vi "Test.vi"() -> ()   [LabVIEW 2020]
uses:
  Classes/KD Tree/KD Tree.lvclass
  Classes/KD Tree Double/Create KD Tree Double.vi
  Classes/KD Tree Double/KD Tree Double.lvclass
  <vilib>/Analysis/NI_AALBase.lvlib
  Classes/KD Tree Double/Find Nearest Neighbors Index Double.vi
  E:/Labview/LV 2020/Schmiedeteilvermessung/Source/libs/SK Spatial/flann/Classes/KD Tree/KD Tree.lvclass
  E:/Labview/LV 2020/Schmiedeteilvermessung/Source/libs/SK Spatial/flann/Classes/KD Tree Double/KD Tree Double.lvclass
  Classes/KD Tree Double/Radius Search Double.vi
  <vilib>/numeric/Random Number (Range) I64.vi
  <vilib>/Analysis/baseanly.llb/Mean (DBL).vi
  flann/Flann Params.ctl
  KD Tree.lvlib
panel:
  out "x/y":dbl
  out "mean":dbl format="%0.2f"
  in  "flann_params 2":T1={"algorithm"=0, "checks"=0, "eps"=0.0, "sorted"=1, "max_neighbors"=-1, "cores"=0, "trees"=0, "leaf_max_size"=0, "branching"=0, "iterations"=0, "centers_init"=0, "cb_index"=0.0, "target_precision"=0.0, "build_weight"=0.0, "memory_weight"=0.0, "sample_fraction"=0.0, "table_number_"=0, "key_size_"=0, "multi_probe_level_"=0, "log_level"=0, "random_seed"=0} {"algorithm" items=["FLANN_INDEX_LINEAR"=0, "FLANN_INDEX_KDTREE"=1, "FLANN_INDEX_KMEANS"=2, "FLANN_INDEX_COMPOSITE"=3, "FLANN_INDEX_KDTREE_SINGLE"=4, "FLANN_INDEX_HIERARCHICAL"=5, "FLANN_INDEX_LSH"=6, "FLANN_INDEX_SAVED"=254, "FLANN_INDEX_AUTOTUNED"=255]; "centers_init" items=["FLANN_CENTERS_RANDOM", "FLANN_CENTERS_GONZALES", "FLANN_CENTERS_KMEANSPP", "FLANN_CENTERS_GROUPWISE"]; "log_level" items=["FLANN_LOG_NONE", "FLANN_LOG_FATAL", "FLANN_LOG_ERROR", "FLANN_LOG_WARN", "FLANN_LOG_INFO", "FLANN_LOG_DEBUG"]}
  out "Ref 2":u64
  out "Ref":u64
  out "P4":dbl[][](array[numeric])
  out "Array":dbl[](array[numeric])
  out "Histogram Graph":T2(graph)
  out "P1":dbl[][](array[numeric])
  out "P2":dbl[][](array[numeric])
  out "Intensity Graph":dbl[][](graph)
  in  "flann_params":T1={"algorithm"=0, "checks"=0, "eps"=0.0, "sorted"=1, "max_neighbors"=-1, "cores"=0, "trees"=0, "leaf_max_size"=0, "branching"=0, "iterations"=0, "centers_init"=0, "cb_index"=0.0, "target_precision"=0.0, "build_weight"=0.0, "memory_weight"=0.0, "sample_fraction"=0.0, "table_number_"=0, "key_size_"=0, "multi_probe_level_"=0, "log_level"=0, "random_seed"=0} {"algorithm" items=["FLANN_INDEX_LINEAR"=0, "FLANN_INDEX_KDTREE"=1, "FLANN_INDEX_KMEANS"=2, "FLANN_INDEX_COMPOSITE"=3, "FLANN_INDEX_KDTREE_SINGLE"=4, "FLANN_INDEX_HIERARCHICAL"=5, "FLANN_INDEX_LSH"=6, "FLANN_INDEX_SAVED"=254, "FLANN_INDEX_AUTOTUNED"=255]; "centers_init" items=["FLANN_CENTERS_RANDOM", "FLANN_CENTERS_GONZALES", "FLANN_CENTERS_KMEANSPP", "FLANN_CENTERS_GROUPWISE"]; "log_level" items=["FLANN_LOG_NONE", "FLANN_LOG_FATAL", "FLANN_LOG_ERROR", "FLANN_LOG_WARN", "FLANN_LOG_INFO", "FLANN_LOG_DEBUG"]}
  out "error out":errorcluster
  out "N Found":i32[](array[numeric])
  out "Dists 2":dbl[][](array[numeric])
  out "Indices 2":i32[][](array[numeric])
  out "Dists":dbl[][](array[numeric])
  out "Indices":i32[][](array[numeric])
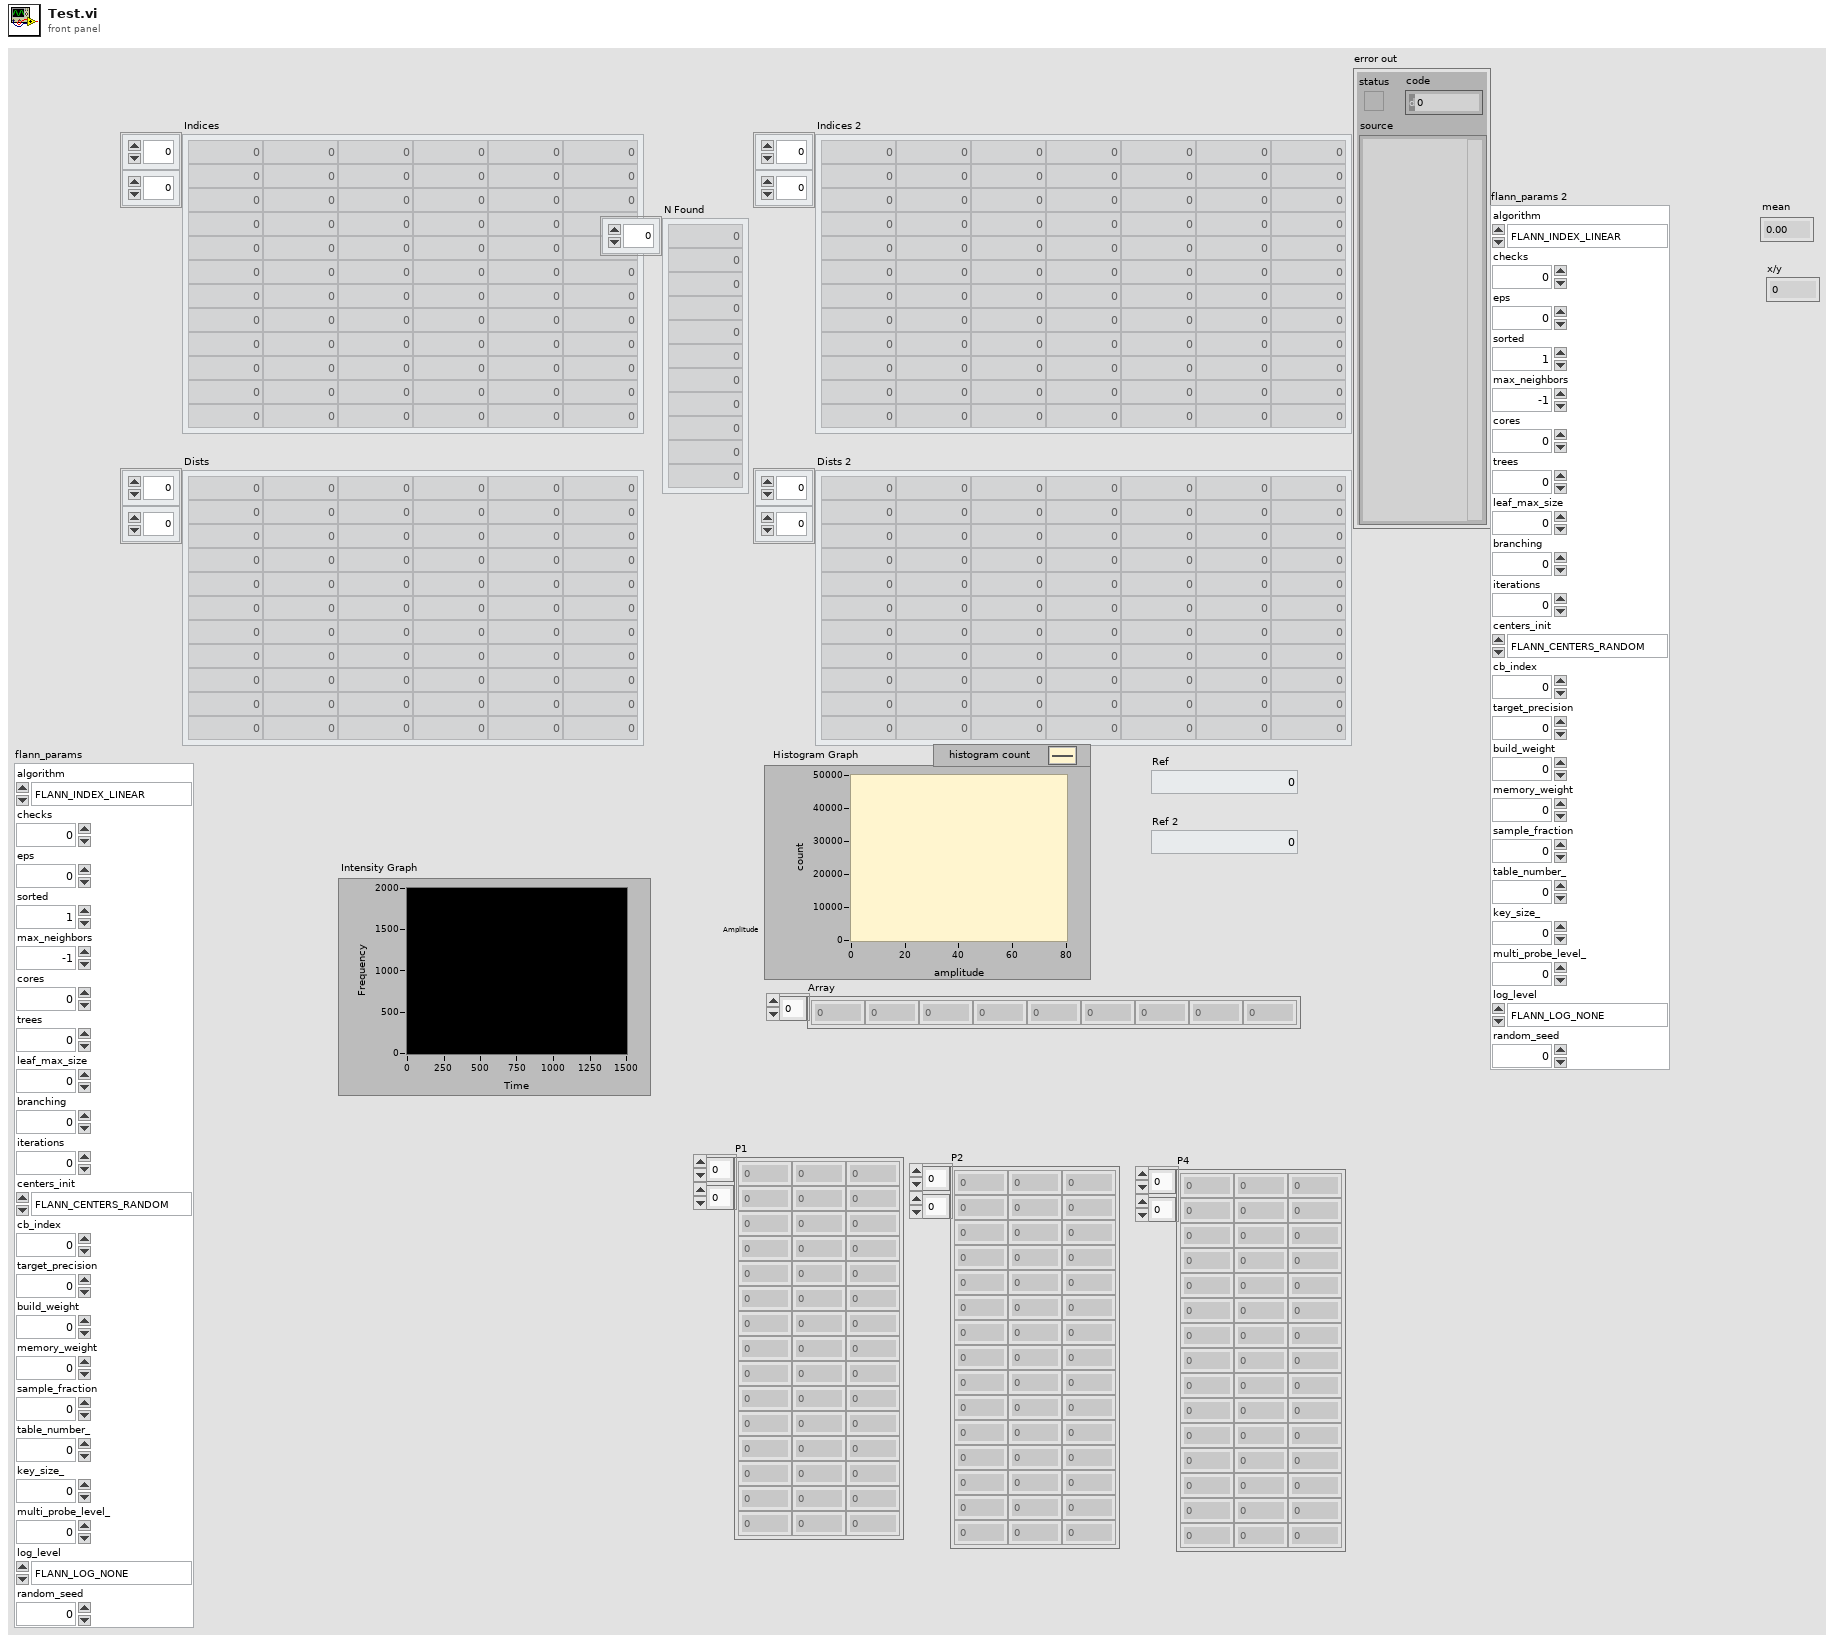
[diagram p1: front panel]
types:
  T1 = typedef "KD Tree.lvlib/Flann Params.ctl" = cluster{"algorithm":u32, "checks":i32, "eps":sgl, "sorted":i32, "max_neighbors":i32, "cores":i32, "trees":i32, "leaf_max_size":i32, "branching":i32, "iterations":i32, "centers_init":u32, "cb_index":sgl, "target_precision":sgl, "build_weight":sgl, "memory_weight":sgl, "sample_fraction":sgl, "table_number_":u32, "key_size_":u32, "multi_probe_level_":u32, "log_level":u32, "random_seed":i32}
  T2 = cluster{"X Values":dbl[], "Histogram: h(x)":i32[]}
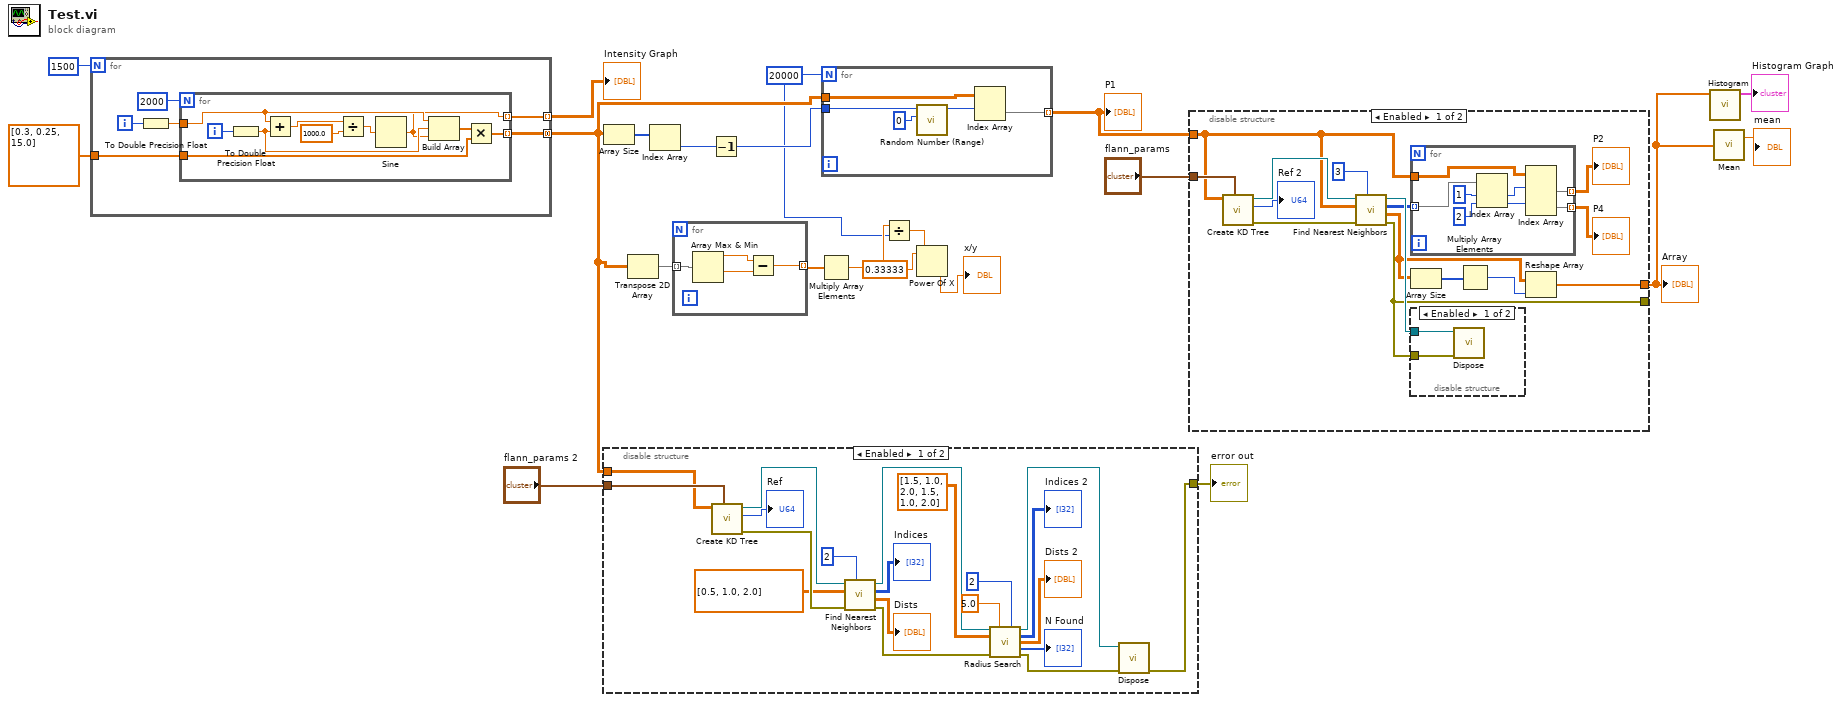
[diagram p0: block diagram]
diagram:
  w4 = 20000
  n1 = for {
    N: 1500 -> [_]
    tunnel: [w27] -> w8 mode=concatenating
    tunnel: [w23] -> w16 mode=indexing
    tunnel: dbl[] [0.3, 0.25, 15.0] ("appended array") -> [w22]
    i -> [w26]
    n2 = To Double Precision Float(number=w26) -> (double precision float=w24:dbl)
    n3 = for {
      N: 2000 -> [_]
      tunnel: [w29] -> w27 mode=indexing
      tunnel: w24 -> [w34]
      tunnel: [w32] -> w23 mode=indexing
      tunnel: w22 -> [w28]
      i -> [w37]
      n4 = To Double Precision Float(number=w37) -> (double precision float=w35:dbl)
      n5 = Add(x=w34, y=w35) -> (x+y=w33:dbl)
      n6 = Divide(x=w33, y=1000.0) -> (x/y=w31:dbl)
      n7 = Sine(x=w31) -> (sin(x)=w32:dbl)
      n8 = Build Array(w34, w35, w32) -> (w36:dbl[])
      n9 = Multiply(x=w36, y=w28) -> (x*y=w29:dbl[])
    }
  }
  "Intensity Graph" <- w16
  n10 = Array Size(array=w8) -> (size(s)=w19:i32[])
  n11 = disable-structure shown="Enabled" {
    disable-tunnel: [w52 _] -> w21
    disable-tunnel: "flann_params 2" -> [w51 _]
    disable-tunnel: w8 -> [w50 _]
    frame Enabled {
      n12 = call-poly "Create KD Tree.vi"("flann_params"=w51, "Points (Row-Vectors)"=w50) -> ("error out"=w47:errorcluster, "Ref"=→"Ref":u64, "KD Tree Double out"=w42:refnum<class "KD Tree Double.lvclass">)  [unwired: 7 in]
      n13 = call-poly "Find Nearest Neighbors.vi"("#Neighbors"=2, "error in (no error)"=w47, "Points"=dbl[][] [[0.5, 1.0, 2.0]], "KD Tree Double in"=w42) -> ("error out"=w46:errorcluster, "Dists"=→"Dists":dbl[][], "Indices"=→"Indices":i32[][], "KD Tree Double out"=w43:refnum<class "KD Tree Double.lvclass">)  [unwired: 4 in]
      n14 = call-poly "Radius Search.vi"("KD Tree Double in"=w43, "Radius"=sgl 5.0, "Max Neighbors"=2, "Points"=dbl[][] [[1.5, 1.0, 2.0], [1.5, 1.0, 2.0]], "error in (no error)"=w46) -> ("KD Tree Double out"=w54:refnum<class "KD Tree Double.lvclass">, "Indices"=→"Indices 2":i32[][], "Dists"=→"Dists 2":dbl[][], "N Found"=→"N Found":i32[], "error out"=w53:errorcluster)  [unwired: 6 in]
      n15 = call "Dispose.vi"("error in (no error)"=w53, "KD Tree in"=w54) -> ("error out"=w52:errorcluster)  [unwired: 9 in]
    }
    frame Disabled {
    }
  }
  "error out" <- w21
  n16 = Transpose 2D Array(2D array=w8) -> (transposed array=w7:dbl[][])
  n17 = Index Array(array=w19) -> (element=w15:i32)  [unwired: 1 in]
  n18 = for {
    tunnel: w7 -> [w61] mode=indexing
    tunnel: [w58] -> w6 mode=indexing
    n19 = Array Max & Min(array=w61) -> (max value=w60:dbl, min value=w59:dbl)  [unwired: 2 out]
    n20 = Subtract(x=w60, y=w59) -> (x-y=w58:dbl)
  }
  n21 = Decrement(x=w15) -> (x-1=w18:i32)
  n22 = Multiply Array Elements(1:w6) -> (0:w5:dbl)
  n23 = for {
    N: w4 -> [_]
    tunnel: w8 -> [w66]
    tunnel: w18 -> [w64]
    tunnel: [w62] -> w13 mode=indexing
    n24 = call-poly <vilib>:"Random Number (Range).vi"("lower bound (-100)"=i64 0, "upper bound (100)"=w64) -> ("number"=w65:i64)  [unwired: 9 in]
    n25 = Index Array(array=w66, index (row)=w65) -> (element=w62:dbl[])  [unwired: 1 in]
  }
  "P1" <- w13
  n26 = Divide(x=w5, y=w4) -> (x/y=w3:dbl)
  n27 = Power Of X(1:w3, 2:0.33333 ("x")) -> (0:→"x/y":dbl)
  n28 = disable-structure shown="Enabled" {
    disable-tunnel: w13 -> [w78 _]
    disable-tunnel: "flann_params" -> [w81 _]
    disable-tunnel: [w71 _] -> w10
    disable-tunnel: [w69 _] -> _
    frame Enabled {
      n29 = call-poly "Create KD Tree.vi"("flann_params"=w81, "Points (Row-Vectors)"=w78) -> ("error out"=w79:errorcluster, "Ref"=→"Ref 2":u64, "KD Tree Double out"=w80:refnum<class "KD Tree Double.lvclass">)  [unwired: 7 in]
      n30 = call-poly "Find Nearest Neighbors.vi"("#Neighbors"=3, "error in (no error)"=w79, "Points"=w78, "KD Tree Double in"=w80) -> ("error out"=w69:errorcluster, "Dists"=w73:dbl[][], "Indices"=w68:i32[][], "KD Tree Double out"=w75:refnum<class "KD Tree Double.lvclass">)  [unwired: 4 in]
      n31 = for {
        tunnel: w78 -> [w91]
        tunnel: [w90] -> w77 mode=indexing
        tunnel: [w89] -> w76 mode=indexing
        tunnel: w68 -> [w88] mode=indexing
        n32 = Index Array(array=w88, index #1=1 ("disabled index (col)"), index #2=2 ("index (col)")) -> (element #1=w85:i32, element #2=w84:i32)
        n33 = Index Array(array=w91, index (row) #1=w85, index (row) #2=w84) -> (element #1=w90:dbl[], element #2=w89:dbl[])  [unwired: 2 in]
      }
      "P2" <- w77
      "P4" <- w76
      n34 = Array Size(array=w73) -> (size(s)=w74:i32[])
      n35 = disable-structure shown="Enabled" {
        disable-tunnel: w75 -> [w83 _]
        disable-tunnel: w69 -> [w82 _]
        frame Enabled {
          n36 = call "Dispose.vi"("error in (no error)"=w82, "KD Tree in"=w83) -> ()  [unwired: 9 in, 1 out]
        }
        frame Disabled {
        }
      }
      n37 = Multiply Array Elements(1:w74) -> (0:w72:i32)
      n38 = Reshape Array(w73, w72) -> (w71:dbl[])
    }
    frame Disabled {
    }
  }
  "Array" <- w10
  n39 = call <vilib>:"Histogram.vi"("X"=w10) -> ("Histogram Graph"=→"Histogram Graph":T2)  [unwired: 7 in, 3 out]
  n40 = call-poly <vilib>:"Mean.vi"("X"=w10) -> ("mean"=→"mean":dbl)  [unwired: 1 out]
